vi "Update Project Tree.vi"(8 "error in (no error)":errorcluster, 11 "Editor.lvclass in":refnum<data-value>) -> (0 "error out":errorcluster, 3 "Editor.lvclass out":refnum<data-value>)   [LabVIEW 2015, in "Editor.lvclass"]
uses:
  Editor.lvclass
  Project.lvclass
  Step.lvclass
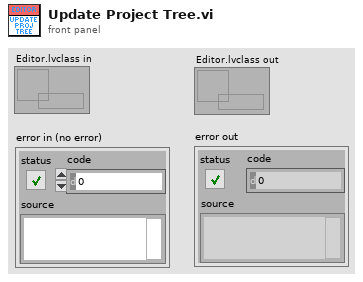
[diagram p1: front panel]
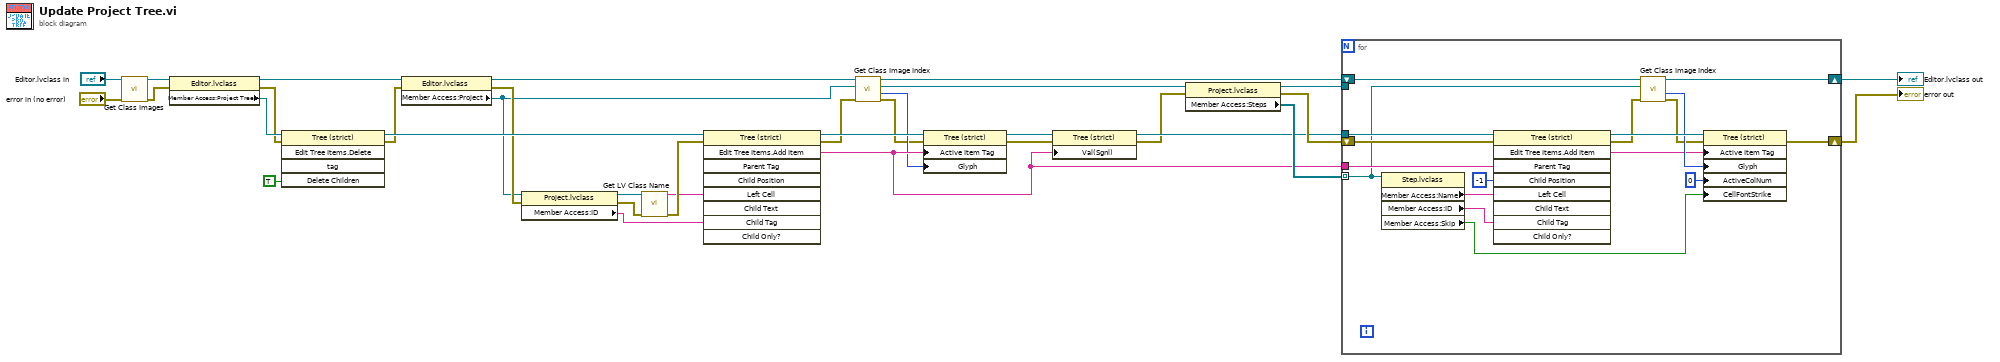
[diagram p0: block diagram]
diagram:
  n1 = call "Get Class Images.vi"("error in (no error)"="error in (no error)", "Editor.lvclass in"="Editor.lvclass in") -> ("error out"=w14:errorcluster, "Editor.lvclass out"=w15:refnum<data-value>)  [unwired: 8 in]
  n2 = property class="Editor.lvclass"(reference=w15, error in=w14) -> (reference out=w11:refnum<data-value>, error out=w12:errorcluster, "Member Access:Project Tree"=w17:refnum<vi>)
  n3 = invoke class="Tree (strict)" method="Edit Tree Items.Delete"(reference=w17, error in=w12, "Delete Children"=TRUE) -> (reference out=w18:refnum<vi>, error out=w10:errorcluster)  [unwired: 2 in, 3 out]
  n4 = property class="Editor.lvclass"(reference=w11, error in=w10) -> (reference out=w8:refnum<data-value>, error out=w9:errorcluster, "Member Access:Project"=w6:refnum<class "Project.lvclass">)
  n5 = property class="Project.lvclass"(reference=w6, error in=w9) -> (reference out=w26:refnum<class "Project.lvclass">, error out=w25:errorcluster, "Member Access:ID"=w24:string)
  n6 = call <vilib>:"Get LV Class Name.vi"("error in (no error)"=w25, "object"=w26) -> ("error out"=w33:errorcluster, "class name"=w19:string)  [unwired: 8 in]
  n7 = invoke class="Tree (strict)" method="Edit Tree Items.Add Item"(reference=w18, error in=w33, "Left Cell"=w19, "Child Tag"=w24) -> (reference out=w23:refnum<vi>, error out=w7:errorcluster, "Edit Tree Items:Add Item"=w22:string)  [unwired: 5 in, 6 out]
  n8 = call "Get Class Image Index.vi"("error in (no error)"=w7, "SerializableObject in"=w6, "Editor.lvclass in"=w8) -> ("error out"=w4:errorcluster, "Index"=w5:i32, "SerializableObject out"=w3:refnum<class "Project.lvclass">, "Editor.lvclass out"=w2:refnum<data-value>)  [unwired: 5 in]
  n9 = property class="Tree (strict)"(reference=w23, error in=w4, "Active Item Tag"=w22, "Glyph"=w5) -> (reference out=w21:refnum<vi>, error out=w20:errorcluster)
  n10 = property class="Tree (strict)"(reference=w21, error in=w20, "Val(Sgnl)"=w22) -> (reference out=w28:refnum<vi>, error out=w27:errorcluster)
  n11 = property class="Project.lvclass"(reference=w3, error in=w27) -> (reference out=w30:refnum<class "Project.lvclass">, error out=w31:errorcluster, "Member Access:Steps"=w32:refnum<class "Step.lvclass">[])
  n12 = for {
    tunnel: w32 -> [w42] mode=indexing
    tunnel: w28 -> [w51]
    tunnel: w30 -> [_]
    shift-right: [w37] -> w29
    shift-left: w31 -> [w50]
    tunnel: w22 -> [w48]
    shift-right: [w39] -> w1
    shift-left: w2 -> [w44]
    n13 = property class="Step.lvclass"(reference=w42) -> ("Member Access:Name"=w49:string, "Member Access:ID"=w47:string, "Member Access:Skip"=w35:bool)  [unwired: 1 in, 2 out]
    n14 = invoke class="Tree (strict)" method="Edit Tree Items.Add Item"(reference=w51, error in=w50, "Parent Tag"=w48, "Child Position"=-1, "Left Cell"=w49, "Child Tag"=w47) -> (reference out=w46:refnum<vi>, error out=w41:errorcluster, "Edit Tree Items:Add Item"=w38:string)  [unwired: 3 in, 6 out]
    n15 = call "Get Class Image Index.vi"("error in (no error)"=w41, "SerializableObject in"=w42, "Editor.lvclass in"=w44) -> ("error out"=w40:errorcluster, "Index"=w43:i32, "Editor.lvclass out"=w39:refnum<data-value>)  [unwired: 5 in, 1 out]
    n16 = property class="Tree (strict)"(reference=w46, error in=w40, "Active Item Tag"=w38, "Glyph"=w43, "ActiveColNum"=0 ("Active Cell:Active Column Number"), "CellFontStrike"=w35) -> (error out=w37:errorcluster)  [unwired: 1 out]
  }
  "error out" <- w29
  "Editor.lvclass out" <- w1
